vi "test_fpga_ort_find_max.vi"() -> ()   [LabVIEW 2016]
uses:
  <vilib>/Platform/TimedLoop/XDataNode/timing_clust.ctl
  <vilib>/Platform/TimedLoop/XDataNode/nitl_modes.ctl
  <vilib>/Platform/TimedLoop/XDataNode/wakeup.ctl
  <vilib>/rvi/Emulation/niFpgaSctlEmulationGetInTimedLoop.vi
  <vilib>/rvi/Emulation/niFpgaEmulationReportErrorSimple.vi
  <vilib>/rvi/Emulation/niFpgaGetClockAttributes.vi
  <vilib>/rvi/Emulation/niFpgaCriticalErrorInLSC.vi
  <vilib>/Platform/TimedLoop/XDataNode/XDataNode.xnode
  <vilib>/Platform/TimedLoop/XDataNode/XDNodeRunTimeDep.lvlib
panel:
  out "cycleMax":fxp<+/-,24,16>
  out "maxIndex":u16
  out "cycleMaxMonitor":fxp<+/-,24,16>
  out "outputValid":bool
  in  "data":cluster{"index":u16, "data":i16}
  in  "ort.p.methodParams":T1
  in  "endOfCycle":bool
  in  "inputValid":bool
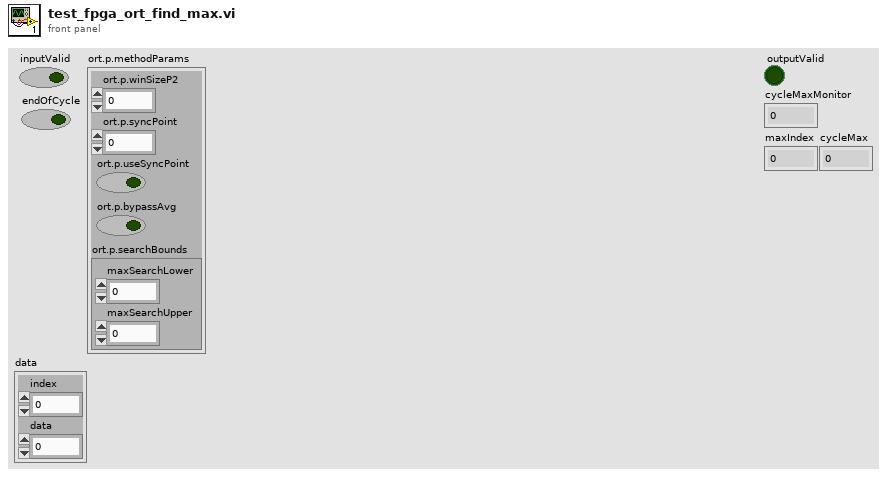
[diagram p1: front panel]
types:
  T1 = cluster{"ort.p.winSizeP2":u16, "ort.p.syncPoint":u16, "ort.p.useSyncPoint":bool, "ort.p.bypassAvg":bool, "ort.p.searchBounds":cluster{"maxSearchLower":u16, "maxSearchUpper":u16}}
  T2 = typedef "XDNodeRunTimeDep.lvlib/timing_clust.ctl" = cluster{"Expected End [f-1]":u64, "Actual End [f-1]":u64, "Finished Late? [f-1]":bool, "Expected End [i-1]":u64, "Actual End [i-1]":u64, "Finished Late? [i-1]":bool, "Expected Start [i]":u64, "Actual Start [i]":u64, "Expected Start [f]":u64, "Actual Start [f]":u64, "Source Name":string, "Structure Name":string, "Period":i64, "Deadline":i64, "Offset":i64, "Start":i64, "Priority":i32, "Timeout":i32, "Mode":T3, "Wakeup Reason":T4, "Error":errorcluster, "Source Type":string, "Secondary Source Type":string, "Global End Time":u64, "Global Start Time":u64, "Frame Duration":u64, "Iteration Duration":u64, "Assigned CPU":i32, "I/O Scan Engine Mode":u32}
  T3 = typedef "XDNodeRunTimeDep.lvlib/nitl_modes.ctl" = enum32{"No Change", "Process missed periods, maintain original phase", "Discard missed periods, maintain original phase", "Process missed periods, ignore original phase", "Discard missed periods, ignore original phase"}
  T4 = typedef "XDNodeRunTimeDep.lvlib/wakeup.ctl" = enum32{"Normal", "Aborted", "Asynchronous wakeup", "Timing source error", "Timed loop error", "Timeout"}
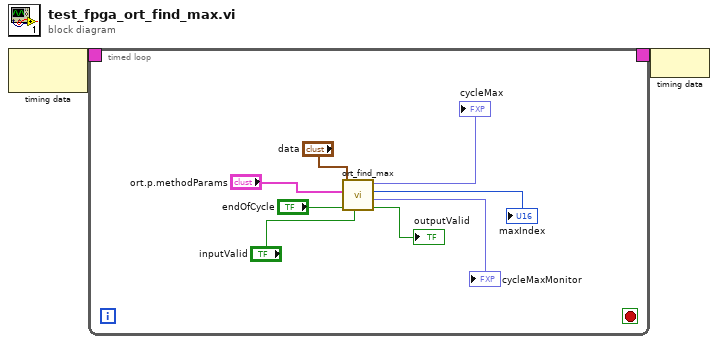
[diagram p0: block diagram]
diagram:
  n1 = node-c288() -> (w2:T2)  [unwired: 1 in]
  n2 = timed-loop {
    timing: w2 -> [_]
    timing-out: [_] -> w1
    stop <- _ stop-if-true
    n3 = call "ort_find_max.vi"("inputValid"="inputValid", "endOfCycle"="endOfCycle", "ort.p.methodParams"="ort.p.methodParams", "data"="data") -> ("outputValid"=→"outputValid":bool, "cycleMaxMonitor"=→"cycleMaxMonitor":fxp<+/-,24,16>, "maxIndex"=→"maxIndex":u16, "cycleMax"=→"cycleMax":fxp<+/-,24,16>)  [unwired: 4 in]
  }
  n4 = node-c288(w1) -> ()
